vi "InsertSocket.vi"() -> ()   [LabVIEW 2012]
uses:
  <vilib>/addons/database/Connection.llb/DB Tools Open Connec (Path).vi
  <vilib>/addons/database/Connection.llb/Conn Execute.vi
  <vilib>/addons/database/Recordset.llb/Rec Fetch Recordset Data (R).vi
  <vilib>/addons/database/Recordset.llb/Rec Destroy - Connection.vi
  <vilib>/addons/database/Recordset.llb/Rec Fetch Integer Data (R).vi
  <vilib>/addons/database/_DB Variant To Data/Database Variant To Data.xnode
  <vilib>/addons/database/NI_Database_API.lvlib
panel:
  out "error out 4":errorcluster
  out "data":i32
  out "concatenated string":string
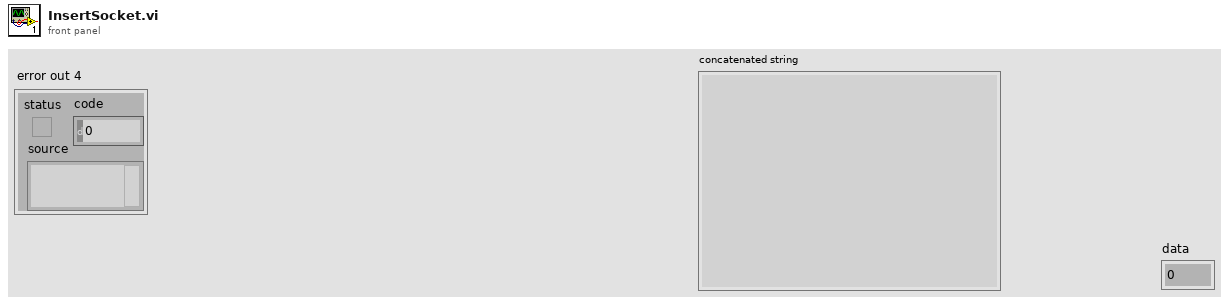
[diagram p1: front panel]
types:
  T1 = typedef "NI_Database_API.lvlib/Conn ObjectReference.ctl" = refnum<k1>
  T2 = typedef "NI_Database_API.lvlib/Rec ObjectReference.ctl" = refnum<k1>
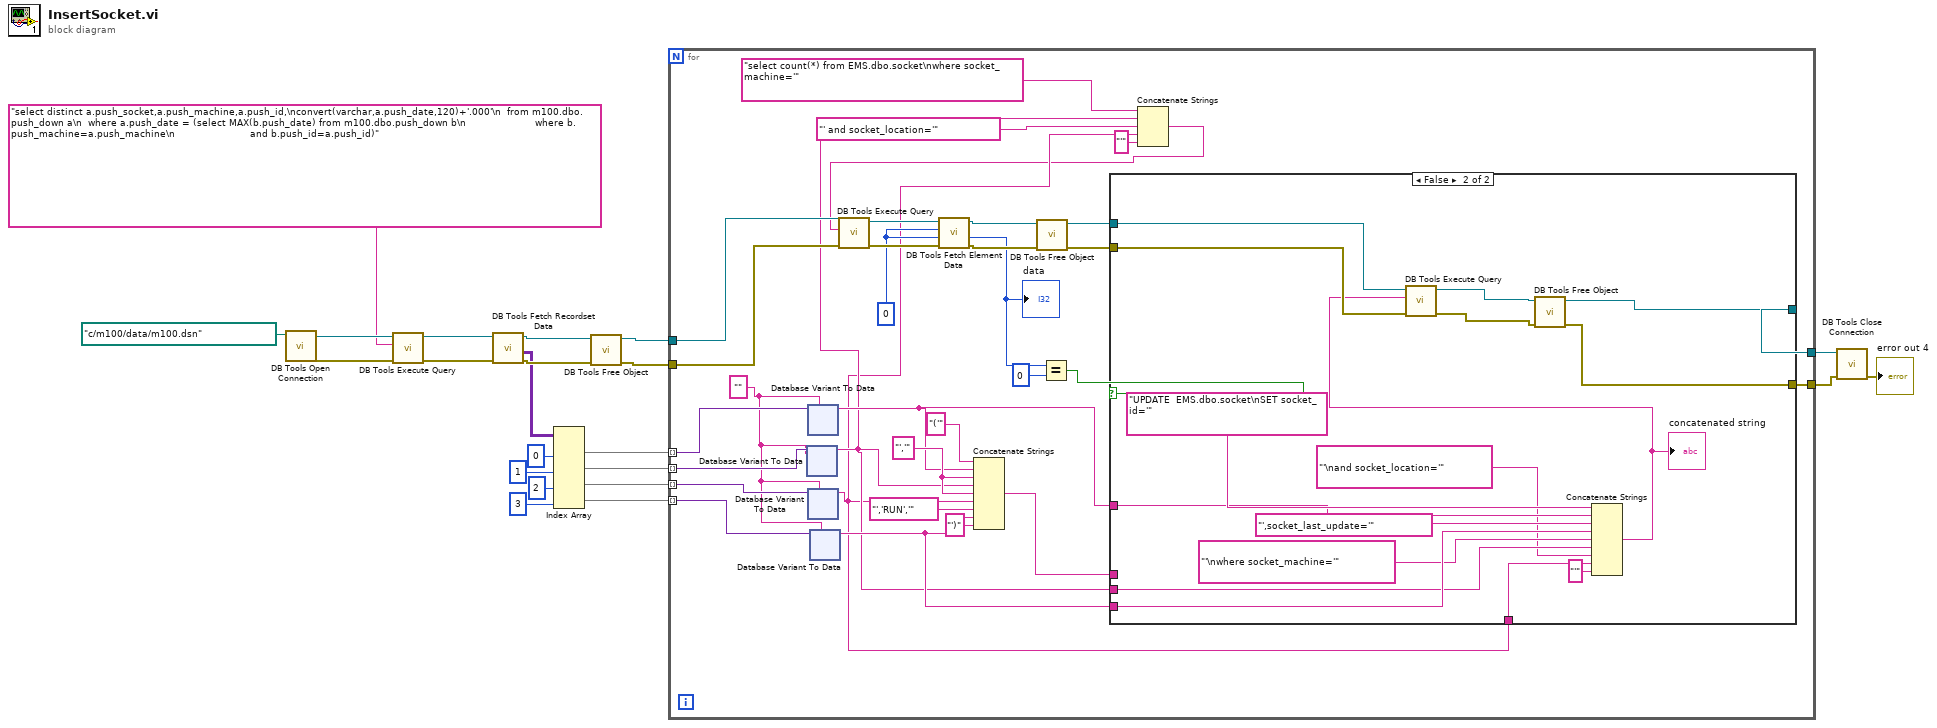
[diagram p0: block diagram]
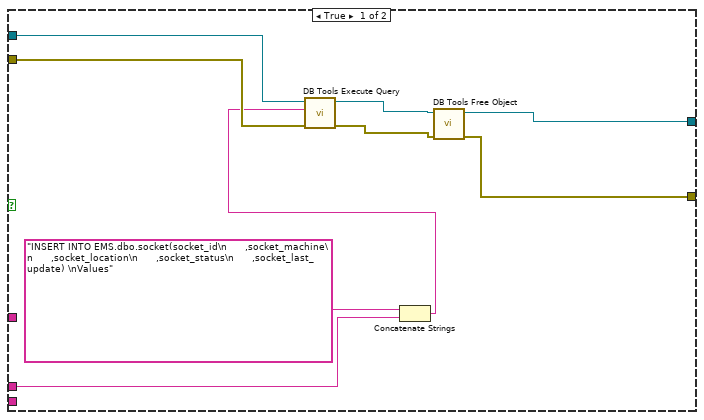
[diagram p2: hidden frame]
diagram:
  n1 = call-poly <vilib>:"DB Tools Open Connection.vi"("connection information"=path "c:/m100/data/m100.dsn") -> ("error out"=w20:errorcluster, "connection reference"=w21:T1)  [unwired: 7 in]
  n2 = call-poly <vilib>:"DB Tools Execute Query.vi"("error in (no error)"=w20, "SQL query"="select distinct a.push_socket,a.push_machine,a.push_id,\nconvert(varchar,a.push_date,120)+'.000'\n  from m100.dbo.push_down a\n  where a.push_date = (select MAX(b.push_date) from m100.dbo.push_down b\n                       where b.push_machine=a.push_machine\n                         and b.push_id=a.push_id)", "connection reference"=w21) -> ("error out"=w18:errorcluster, "recordset reference"=w19:T2)  [unwired: 5 in]
  n3 = call-poly <vilib>:"DB Tools Fetch Recordset Data.vi"("error in (no error)"=w18, "recordset reference"=w19) -> ("error out"=w16:errorcluster, "recordset data"=w9:variant[][], "recordset reference out"=w17:T2)  [unwired: 3 in]
  n4 = Index Array(array=w9, index (col) #1=0 ("disabled index (col)"), index (col) #2=1 ("index (col)"), index (col) #3=2 ("index (col)"), index (col) #4=3 ("index (col)")) -> (element #1=w4:variant[], element #2=w3:variant[], element #3=w2:variant[], element #4=w1:variant[])  [unwired: 4 in]
  n5 = call-poly <vilib>:"DB Tools Free Object.vi"("error in (no error)"=w16, "recordset reference"=w17) -> ("error out"=w14:errorcluster, "connection reference"=w15:T1)  [unwired: 8 in]
  n6 = for {
    tunnel: w15 -> [w42]
    tunnel: w14 -> [w41]
    tunnel: [w32] -> w11
    tunnel: [w31] -> w10
    tunnel: w4 -> [w54] mode=indexing
    tunnel: w3 -> [w53] mode=indexing
    tunnel: w2 -> [w52] mode=indexing
    tunnel: w1 -> [w51] mode=indexing
    w36 = "','" ("string")
    w45 = 0
    w50 = ""
    n7 = xnode "Database Variant To Data"("database variant"=w53, "type"=w50) -> ("data"=w27:string)  [unwired: 1 in, 1 out]
    n8 = xnode "Database Variant To Data"("database variant"=w54, "type"=w50) -> ("data"=w30:string)  [unwired: 1 in, 1 out]
    n9 = xnode "Database Variant To Data"("database variant"=w52, "type"=w50) -> ("data"=w25:string)  [unwired: 1 in, 1 out]
    n10 = xnode "Database Variant To Data"("database variant"=w51, "type"=w50) -> ("data"=w29:string)  [unwired: 1 in, 1 out]
    n11 = Concatenate Strings("('" ("string"), w30, w36, w27, w36, w25, "','RUN','" ("string"), w29, "')" ("string")) -> (w33:string)
    n12 = Concatenate Strings("select count(*) from EMS.dbo.socket\nwhere socket_machine='" ("SQL query"), w27, "' and socket_location='" ("string"), w25, "'" ("string")) -> (w23:string)
    n13 = call-poly <vilib>:"DB Tools Execute Query.vi"("error in (no error)"=w41, "SQL query"=w23, "connection reference"=w42) -> ("error out"=w48:errorcluster, "recordset reference"=w49:T2)  [unwired: 5 in]
    n14 = call-poly <vilib>:"DB Tools Fetch Element Data.vi"("error in (no error)"=w48, "type"=w45, "column index"=w45, "recordset reference"=w49) -> ("error out"=w46:errorcluster, "data"=w44:i32, "recordset reference out"=w47:T2)  [unwired: 3 in]
    "data" <- w44
    n15 = call-poly <vilib>:"DB Tools Free Object.vi"("error in (no error)"=w46, "recordset reference"=w47) -> ("error out"=w38:errorcluster, "connection reference"=w39:T1)  [unwired: 8 in]
    n16 = Equal?(x=w44, y=0) -> (x = y?=w40:bool)
    n17 = case shown="False" w40 {
      tunnel: w39 -> [w63 w79]
      tunnel: w38 -> [w62 w78]
      tunnel: w33 -> [w61 _]
      tunnel: [w56 w73] -> w32
      tunnel: [w55 w72] -> w31
      tunnel: w30 -> [_ w71]
      tunnel: w29 -> [_ w69]
      tunnel: w27 -> [_ w67]
      tunnel: w25 -> [_ w65]
      frame True {
        n18 = Concatenate Strings("INSERT INTO EMS.dbo.socket(socket_id\n      ,socket_machine\n      ,socket_location\n      ,socket_status\n      ,socket_last_update) \nValues" ("SQL query"), w61) -> (w59:string)
        n19 = call-poly <vilib>:"DB Tools Execute Query.vi"("error in (no error)"=w62, "SQL query"=w59, "connection reference"=w63) -> ("error out"=w57:errorcluster, "recordset reference"=w58:T2)  [unwired: 5 in]
        n20 = call-poly <vilib>:"DB Tools Free Object.vi"("error in (no error)"=w57, "recordset reference"=w58) -> ("error out"=w55:errorcluster, "connection reference"=w56:T1)  [unwired: 8 in]
      }
      frame False {
        n21 = Concatenate Strings("UPDATE  EMS.dbo.socket\nSET socket_id='" ("SQL query"), w71, "',socket_last_update='" ("string"), w69, "'\nwhere socket_machine='" ("string"), w67, "'\nand socket_location='" ("string"), w65, "'" ("string")) -> (w76:string)
        "concatenated string" <- w76
        n22 = call-poly <vilib>:"DB Tools Execute Query.vi"("error in (no error)"=w78, "SQL query"=w76, "connection reference"=w79) -> ("error out"=w74:errorcluster, "recordset reference"=w75:T2)  [unwired: 5 in]
        n23 = call-poly <vilib>:"DB Tools Free Object.vi"("error in (no error)"=w74, "recordset reference"=w75) -> ("error out"=w72:errorcluster, "connection reference"=w73:T1)  [unwired: 8 in]
      }
    }
  }
  n24 = call <vilib>:"DB Tools Close Connection.vi"("error in (no error)"=w10, "connection reference"=w11) -> ("error out"=→"error out 4":errorcluster)  [unwired: 5 in]
